vi "Measurement UI.vi"() -> ()   [LabVIEW 2021, in "Efficiency_Channel Ganging.lvlib"]
uses:
  Efficiency_Channel Ganging.lvlib
panel:
  in  "MeasGraphs":enum32{"Efficiency", "Hidden Controls"}(tab)
  out "EfficiencyGraph":T1(graph)
  in  "Load slave resource names":string[](array[string])
  in  "Load master resouce name":string
  in  "Source slave resource names":string[](array[string])
  in  "Source master resouce name":string
  out "Load sweep points":i32
  out "Source sweep points":i32
  out "Voltage values":dbl[](array[numeric])
  out "Efficiency":dbl[](array[numeric])
  out "Ganged load currents":dbl[](array[numeric])
  in  "MeasConfigurations":T2(tab)=enum."Source Config"
  in  "Source delay":dbl=0.005 caption="SOURCE DELAY" format="%.3ps"
  in  "DUT setup time":dbl=1.0 caption="DUT SETUP TIME" format="%.3ps"
  in  "Aperture time":dbl=0.005 caption="APERTURE TIME" format="%.3ps"
  in  "PPSSlaveResourceNames":refnum<k15>[](array[refnum]) caption="SLAVE RESOURCE NAMES"
  in  "PPSMasterResourceName":refnum<k15> caption="MASTER RESOURCE NAME"
  in  "Source stop voltage":dbl=14.0 caption="VOLTAGE STOP LEVEL" format="%#_6pV"
  in  "Source transient response":i32(ring)=1038 caption="TRANSIENT RESPONSE" items=["Slow"=1041, "Normal"=1038, "Fast"=1039]
  in  "Source sense":i32(ring)=1009 caption="SENSE" items=["Local"=1008, "Remote"=1009]
  in  "Source voltage level range":dbl=20.0 caption="VOLTAGE LEVEL RANGE" format="%#_6pV"
  in  "Source start voltage":dbl=6.0 caption="VOLTAGE START LEVEL" format="%#_6pV"
  in  "Source current limit high":dbl=25.0 caption="CURRENT LIMIT/LIMIT HIGH" format="%#_6pA"
  in  "Source current limit range":dbl=25.0 caption="CURRENT LIMIT RANGE" format="%#_6pA"
  in  "Source limit symmetry":enum32{"Symmetric", "Asymmetric"}(ring)=enum."Asymmetric" caption="LIMIT SYMMETRY"
  in  "Source current limit low":dbl=-0.6 caption="CURRENT LIMIT LOW" format="%#_6pA"
  in  "Source system configuration":enum32{"Series", "Parallel"}(ring)=enum."Parallel" caption="SYSTEM CONFIG"
  in  "Source compliance":string="Compliance"
  in  "Source sourceadapt":string="SourceAdapt"
  in  "Source voltage sweep points":i32=4 caption="NO. OF POINTS"
  in  "Load current sweep points/points per decade":i32=10 caption="PTS/PTS PER DECADE"
  in  "Load sweep type":string(combo)="Logarithmic" caption="SWEEP TYPE"
  in  "Load stop current":dbl=50.0 caption="CURRENT STOP LEVEL" format="%#_6pA"
  in  "Load sourceadapt":string="SourceAdapt"
  in  "Load compliance":string="Compliance"
  in  "Load system configuration":enum32{"Series", "Parallel"}(ring)=enum."Parallel" caption="SYSTEM CONFIG"
  in  "Load voltage limit low":dbl caption="VOLTAGE  LIMIT LOW" format="%#_6pV"
  in  "Load limit symmetry":enum32{"Symmetric", "Asymmetric"}(ring) caption="LIMIT SYMMETRY"
  in  "Load voltage limit range":dbl=6.0 caption="VOLTAGE LIMIT RANGE" format="%#_6pV"
  in  "Load voltage limit high":dbl=inf caption="VOLTAGE LIMIT/LIMIT HIGH" format="%#_6p"
  in  "Load start current":dbl=2.0 caption="CURRENT START LEVEL" format="%#_6pA"
  in  "Load current level range":dbl=80.0 caption="CURRENT LEVEL RANGE" format="%#_6pA"
  in  "Load sense":i32(ring)=1009 caption="SENSE" items=["Local"=1008, "Remote"=1009]
  in  "Load transient response":i32(ring)=1038 caption="TRANSIENT RESPONSE" items=["Slow"=1041, "Normal"=1038, "Fast"=1039]
  in  "LoadSlaveResourceNames":refnum<k15>[](array[refnum]) caption="SLAVE RESOURCE NAMES"
  in  "LoadMasterResourceName":refnum<k15> caption="MASTER RESOURCE NAME"
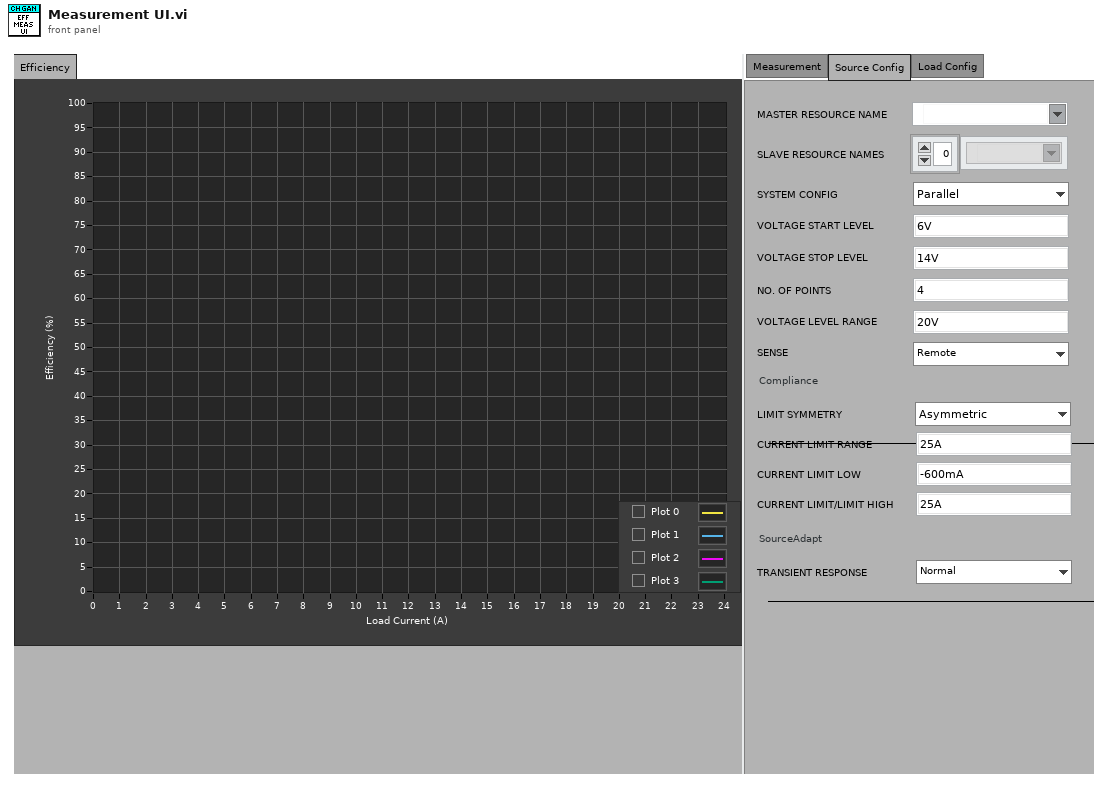
[diagram p1: front panel]
types:
  T1 = cluster{"Ganged load currents":dbl[], "Efficiency":dbl[]}[]
  T2 = enum32{"Measurement", "Source Config", "Load Config"}
  T3 = cluster{"Ganged load currents":dbl[], "Efficiency":dbl[]}
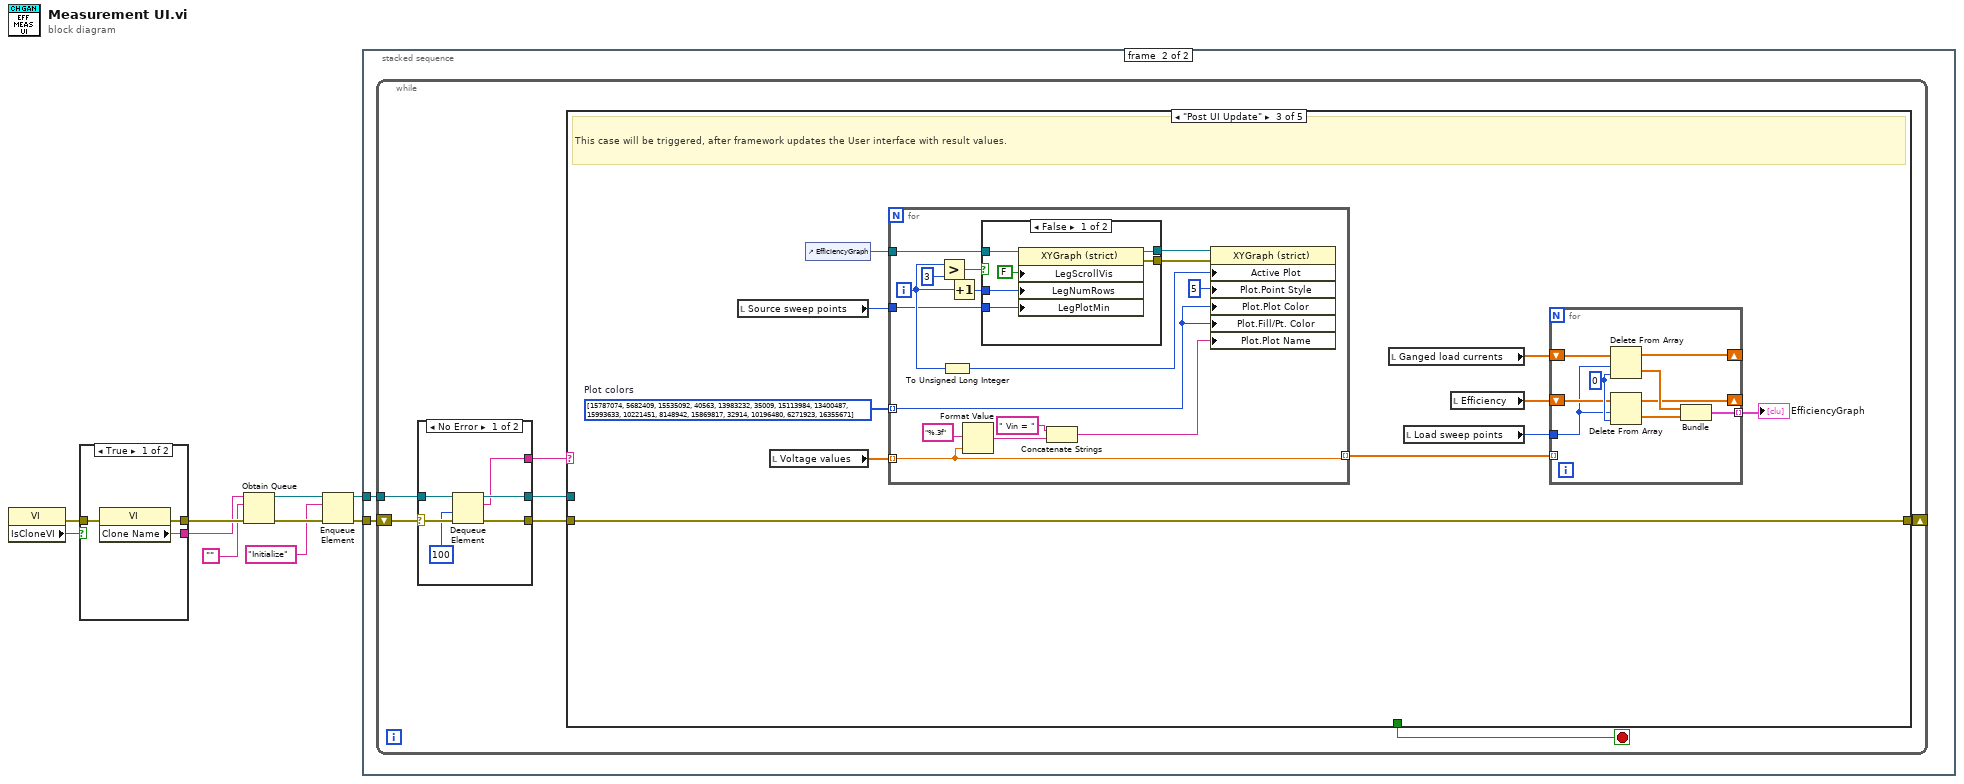
[diagram p0: block diagram]
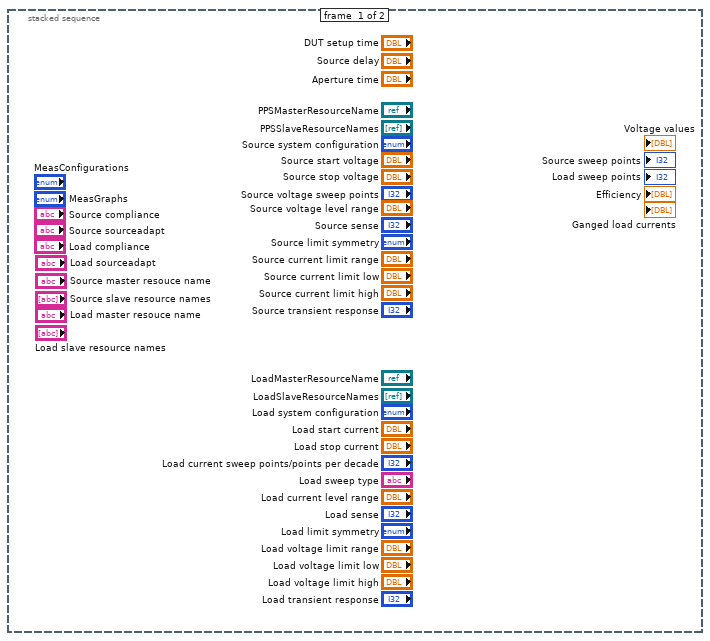
[diagram p2: hidden frame]
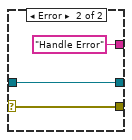
[diagram p3: hidden frame]
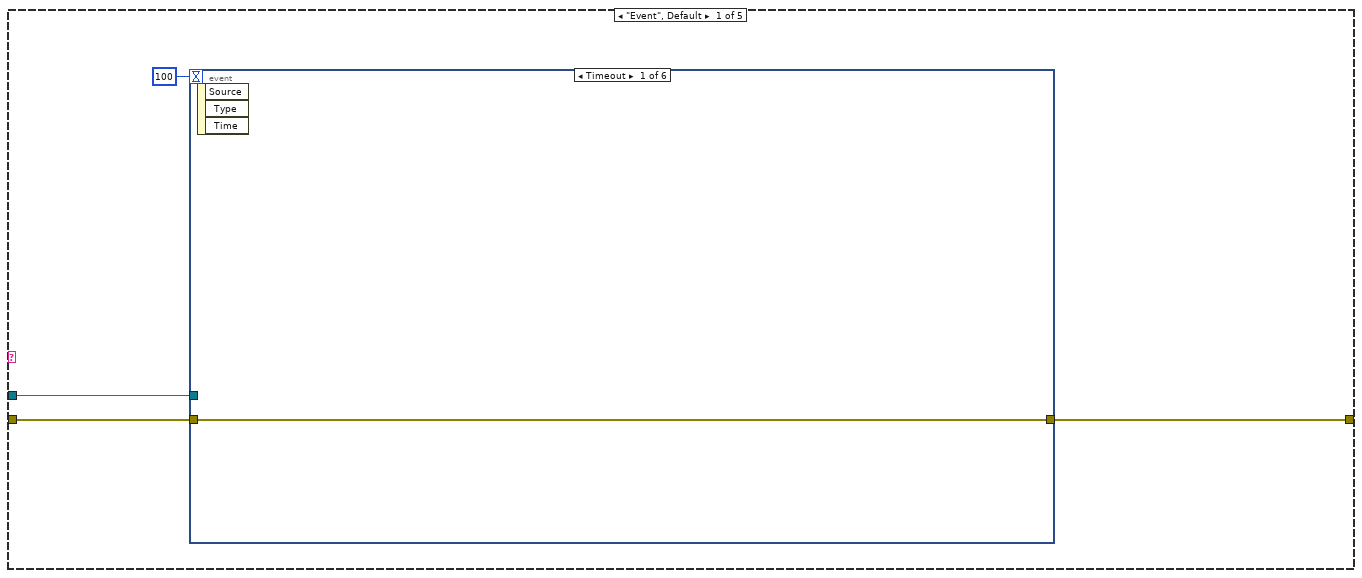
[diagram p4: hidden frame]
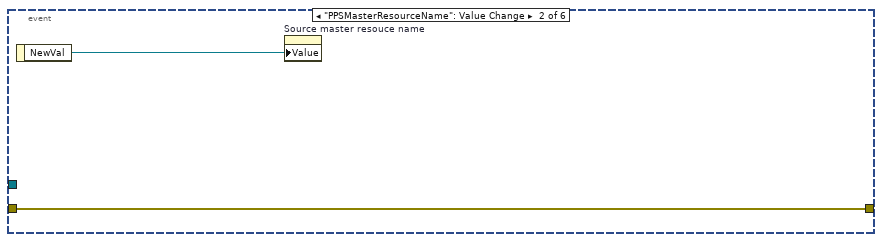
[diagram p5: hidden frame]
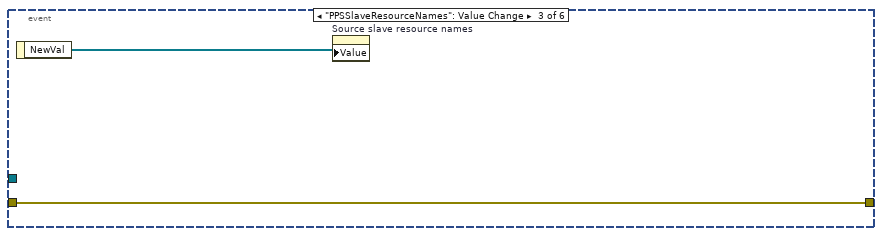
[diagram p6: hidden frame]
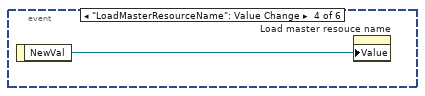
[diagram p7: hidden frame]
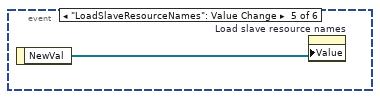
[diagram p8: hidden frame]
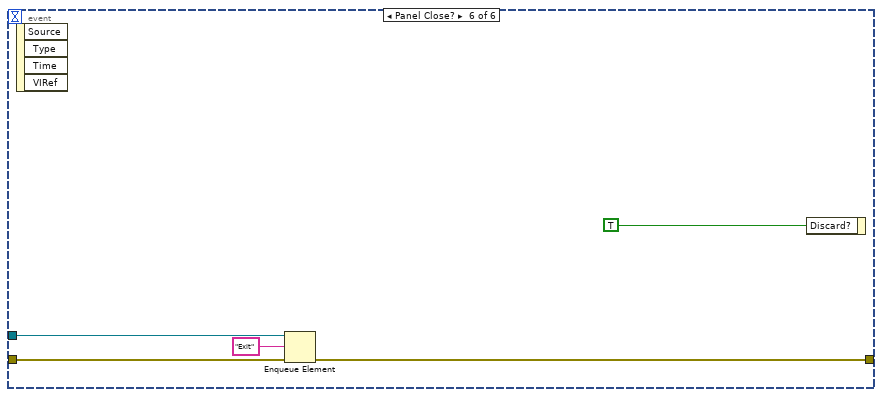
[diagram p9: hidden frame]
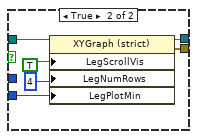
[diagram p11: hidden frame]
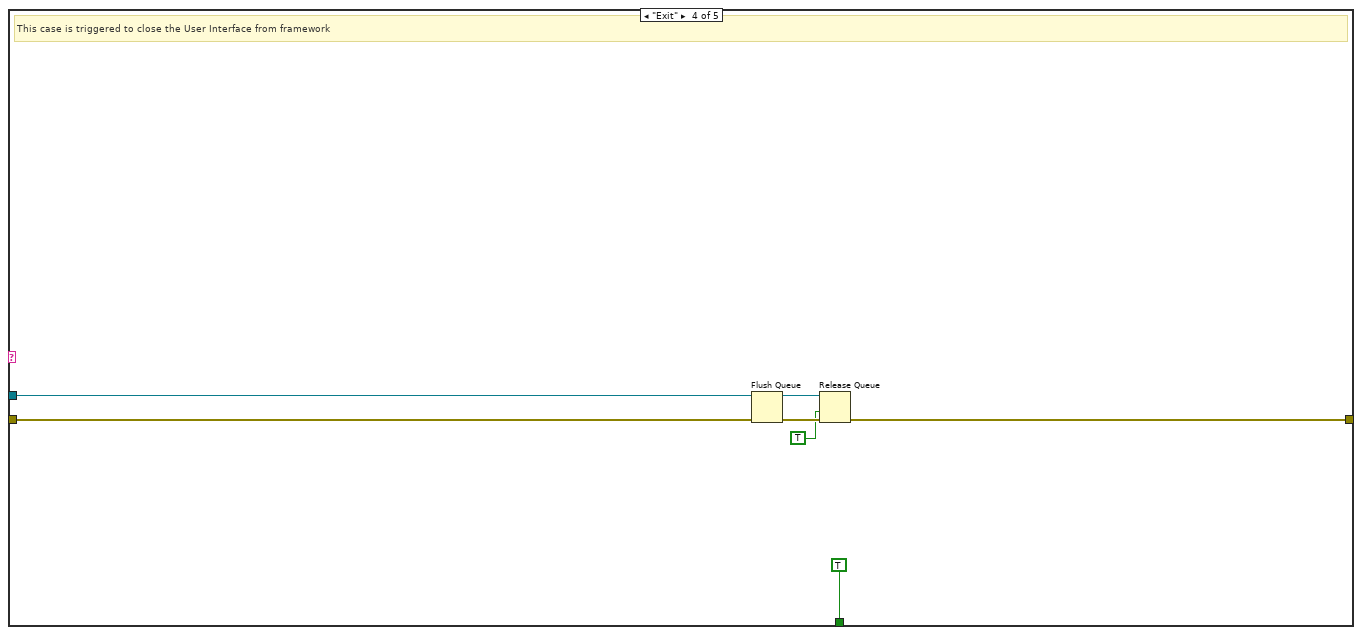
[diagram p12: hidden frame]
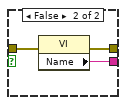
[diagram p14: hidden frame]
diagram:
  n1 = property class="VI"() -> (error out=w1:errorcluster, "IsCloneVI"=w2:bool)  [unwired: 2 in, 1 out]
  n2 = case shown="True" w2 {
    tunnel: [w13 w16] -> w10
    tunnel: [w12 w15] -> w9
    tunnel: w1 -> [w11 w14]
    frame True {
      n3 = property class="VI"(error in=w11) -> (error out=w13:errorcluster, "Clone Name"=w12:string)  [unwired: 1 in, 1 out]
    }
    frame False {
      n4 = property class="VI"(error in=w14) -> (error out=w16:errorcluster, "Name"=w15:string)  [unwired: 1 in, 1 out]
    }
  }
  n5 = Obtain Queue(name (unnamed)=w9, element data type="", error in (no error)=w10) -> (queue out=w6:refnum<queue>, error out=w8:errorcluster)  [unwired: 2 in, 1 out]
  n6 = Enqueue Element(queue=w6, element="Initialize", error in (no error)=w8) -> (queue out=w5:refnum<queue>, error out=w7:errorcluster)  [unwired: 1 in, 1 out]
  n7 = stacked-sequence {
    tunnel: w7 -> [_ w18]
    tunnel: w5 -> [_ w17]
    frame #0 {
    }
    frame #1 {
      n8 = while {
        shift-right: [w20] -> _
        shift-left: w18 -> [w25]
        tunnel: w17 -> [w23]
        stop <- w19 stop-if-true
        n9 = case shown="No Error" w25 {
          selector: w25 -> [w31 w34]
          tunnel: [w30 w34] -> w24
          tunnel: w23 -> [w29 w33]
          tunnel: [w28 w33] -> w22
          tunnel: [w27 "Handle Error"] -> w21
          frame No Error {
            n10 = Dequeue Element(queue=w29, timeout in ms (-1)=100, error in (no error)=w31) -> (queue out=w28:refnum<queue>, element=w27:string, error out=w30:errorcluster)  [unwired: 1 out]
          }
          frame Error {
          }
        }
        n11 = case shown="\"Post UI Update\"" w21 {
          tunnel: w24 -> [w37 w51 w61 w105 w106]
          tunnel: w22 -> [w35 _ _ w103 _]
          tunnel: [w38 w51 w61 w100 w106] -> w20
          tunnel: [_ _ _ TRUE _] -> w19
          frame "Event", Default {
            n12 = event shown="[0] Timeout" {
              selector: _ -> [_ _ _ _ _ _]
              dyn-events: _ -> [_ _ _ _ _ _]
              timeout: 100 -> [_ _ _ _ _ _]
              tunnel: [w39 w41 w43 _ _ w48] -> w38
              tunnel: w37 -> [w39 w41 w43 _ _ w49]
              tunnel: w35 -> [_ _ _ _ _ w47]
              event Timeout {
                n13 = event-data() -> ()  [unwired: 1 in, 3 out]
              }
              event "PPSMasterResourceName": Value Change {
                n14 = event-data() -> ("NewVal"=w40:refnum<k15>)  [unwired: 1 in]
                n15 = property on="Source master resouce name" class="Str"("Value"=w40) -> ()  [unwired: 2 in, 2 out]
              }
              event "PPSSlaveResourceNames": Value Change {
                n16 = event-data() -> ("NewVal"=w42:refnum<k15>[])  [unwired: 1 in]
                n17 = property on="Source slave resource names" class="Arr (strict)"("Value"=w42) -> ()  [unwired: 2 in, 2 out]
              }
              event "LoadMasterResourceName": Value Change {
                n18 = event-data() -> ("NewVal"=w44:refnum<k15>)  [unwired: 1 in]
                n19 = property on="Load master resouce name" class="Str"("Value"=w44) -> ()  [unwired: 2 in, 2 out]
              }
              event "LoadSlaveResourceNames": Value Change {
                n20 = event-data() -> ("NewVal"=w45:refnum<k15>[])  [unwired: 1 in]
                n21 = property on="Load slave resource names" class="Arr (strict)"("Value"=w45) -> ()  [unwired: 2 in, 2 out]
              }
              event Panel Close? {
                n22 = event-data() -> ()  [unwired: 1 in, 4 out]
                n23 = Enqueue Element(queue=w47, element="Exit", error in (no error)=w49) -> (error out=w48:errorcluster)  [unwired: 1 in, 2 out]
                n24 = event-data("Discard?"=TRUE) -> ()  [unwired: 1 in, 1 out]
              }
            }
          }
          frame "Initialize" {
          }
          frame "Post UI Update" {
            w56 = u32[] [15787074, 5682409, 15535092, 40563, 13983232, 35009, 15113984, 13400487, 15993633, 10221451, 8148942, 15869817, 32914, 10196480, 6271923, 16355671]  # Plot colors
            # "This case will be triggered, after framework updates the User interface with result values."
            n25 = local read "Source sweep points"() -> (w53:i32)
            n26 = local read "Voltage values"() -> (w54:dbl[])
            n27 = control-ref of="EfficiencyGraph"() -> (w55:refnum<vi>)
            n28 = for {
              tunnel: w54 -> [w74] mode=indexing
              tunnel: [w74] -> w52 mode=indexing
              tunnel: w55 -> [w67]
              tunnel: w53 -> [w64]
              tunnel: w56 -> [w70] mode=indexing
              i -> [w68]
              n29 = Greater?(x=w68, y=3) -> (0:w72:bool)
              n30 = To Unsigned Long Integer(number=w68) -> (unsigned 32bit integer=w71:u32)
              n31 = Increment(x=w68) -> (x+1=w66:i32)
              n32 = Format Value(format string="%.3f", value (0)=w74) -> (output string=w77:string)  [unwired: 1 out]
              n33 = case shown="False" w72 {
                tunnel: w67 -> [w83 w89]
                tunnel: w66 -> [w82 _]
                tunnel: [w81 w88] -> w65
                tunnel: w64 -> [w79 w84]
                tunnel: [w80 w87] -> w63
                frame False {
                  n34 = property on="Property Node" class="XYGraph (strict)"(reference=w83, "LegScrollVis"=FALSE ("Legend:Scrollbar Visible"), "LegNumRows"=w82, "LegPlotMin"=w79) -> (reference out=w81:refnum<vi>, error out=w80:errorcluster)  [unwired: 1 in]
                }
                frame True {
                  n35 = property on="Property Node" class="XYGraph (strict)"(reference=w89, "LegScrollVis"=TRUE ("Legend:Scrollbar Visible"), "LegNumRows"=u32 4 ("Legend:Number of Rows"), "LegPlotMin"=w84) -> (reference out=w88:refnum<vi>, error out=w87:errorcluster)  [unwired: 1 in]
                }
              }
              n36 = Concatenate Strings(" Vin = " ("string"), w77) -> (w62:string)
              n37 = property on="Property Node" class="XYGraph (strict)"(reference=w65, error in=w63, "Active Plot"=w71, "Plot.Point Style"=u8 5, "Plot.Plot Color"=w70, "Plot.Fill/Pt. Color"=w70, "Plot.Plot Name"=w62) -> ()  [unwired: 2 out]
            }
            n38 = local read "Ganged load currents"() -> (w60:dbl[])
            n39 = local read "Load sweep points"() -> (w57:i32)
            n40 = local read "Efficiency"() -> (w59:dbl[])
            n41 = for {
              tunnel: [w98] -> w58 mode=indexing
              shift-right: [w97] -> _
              shift-left: w60 -> [w93]
              shift-right: [w91] -> _
              shift-left: w59 -> [w92]
              tunnel: w57 -> [w90]
              tunnel: w52 -> [_] mode=indexing
              w94 = 0 ("index")
              n42 = Delete From Array(array=w93, length=w90, index=w94) -> (deleted portion=w96:dbl[], array with subset deleted=w97:dbl[])
              n43 = Delete From Array(array=w92, length=w90, index=w94) -> (deleted portion=w95:dbl[], array with subset deleted=w91:dbl[])
              n44 = Bundle("Ganged load currents"=w96, "Efficiency"=w95) -> (w98:T3)  [unwired: 1 in]
            }
            "EfficiencyGraph" <- w58
          }
          frame "Exit" {
            # "This case is triggered to close the User Interface from framework"
            n45 = Flush Queue(queue=w103, error in (no error)=w105) -> (queue out=w102:refnum<queue>, error out=w101:errorcluster)  [unwired: 1 out]
            n46 = Release Queue(queue=w102, force destroy? (F)=TRUE, error in (no error)=w101) -> (error out=w100:errorcluster)  [unwired: 2 out]
          }
          frame "Handle Error" {
          }
        }
      }
    }
  }
